vi "Delete Selected Path from List.vi"(8 "error in (no error)":errorcluster, 11 "ListBox in":refnum<vi>) -> (0 "error out":errorcluster, 3 "ListBox out":refnum<vi>)   [LabVIEW 2013, in "Example Configuration Dialog.lvlib" / "Example Configuration Dialog.lvclass"]
uses:
  Example Configuration Dialog.lvclass
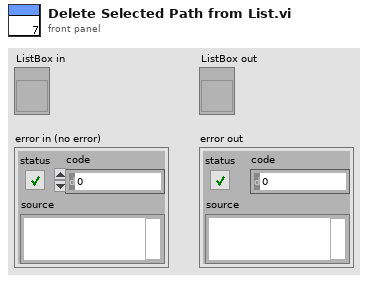
[diagram p1: front panel]
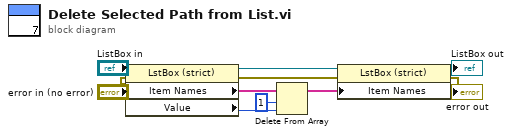
[diagram p0: block diagram]
diagram:
  n1 = property on="Property Node" class="LstBox (strict)"(reference="ListBox in", error in="error in (no error)") -> (reference out=w4:refnum<vi>, error out=w9:errorcluster, "Item Names"=w3:string[], "Value"=w2:i32)
  n2 = Delete From Array(array=w3, length=1, index=w2) -> (array with subset deleted=w6:string[])  [unwired: 1 out]
  n3 = property on="Property Node" class="LstBox (strict)"(reference=w4, error in=w9, "Item Names"=w6) -> (reference out=→"ListBox out":refnum<vi>, error out=→"error out":errorcluster)
